vi "KG set molarity.vi"(7 "Info Cluster":T1, 8 "Fehler (Eingang, kein Fehler)":errorcluster, 9 "molarity":dbl, 10 "pump":u32, 11 "VISA-Ressourcenname":refnum<visa-resource-name>) -> (0 "Fehler (Ausgang)":errorcluster, 2 "Kommando gesendet":string, 3 "VISA-Ressourcenname (Ausgang)":refnum<visa-resource-name>)   [LabVIEW 2020, in "Linearisierung v2.lvlib" / "Gasteiler.lvlib" / "HovaCAL_Interface.lvlib" / "KGN.lvlib" / "set.lvlib"]
uses:
  set.lvlib
  Controls/Info Cluster.ctl
  KGN.lvlib
  Controls/Controls.lvlib
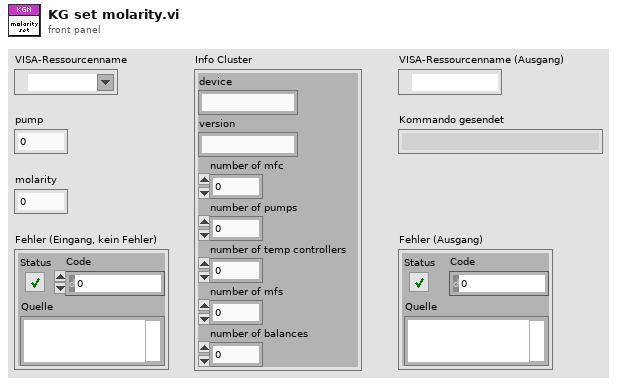
[diagram p1: front panel]
types:
  T1 = typedef "Linearisierung v2.lvlib/Gasteiler.lvlib/HovaCAL_Interface.lvlib/Controls.lvlib/Info Cluster.ctl" = cluster{"device":string, "version":string, "number of mfc":i32, "number of pumps":i32, "number of temp controllers":i32, "number of mfs":i32, "number of balances":i32}
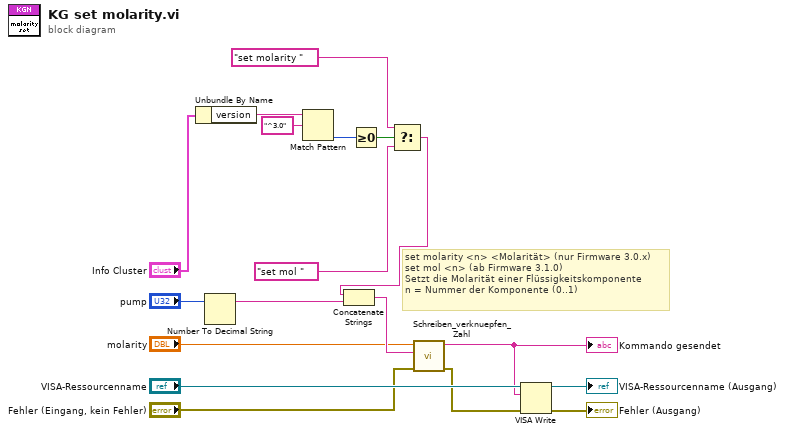
[diagram p0: block diagram]
diagram:
  # "set molarity <n> <Molarität> (nur Firmware 3.0.x)\nset mol <n> (ab Firmware 3.1.0)\nSetzt die Molarität einer Flüssigkeitskomponente\nn = Nummer der Komponente (0..1)"
  n1 = Unbundle By Name("Info Cluster") -> ("version"=w7:string)
  n2 = Number To Decimal String(number="pump") -> (decimal integer string=w14:string)  [unwired: 1 in]
  n3 = Match Pattern(string=w7, regular expression="^3.0" ("Regulärer Ausdruck")) -> (offset past match=w5:i32)  [unwired: 1 in, 3 out]
  n4 = Greater Or Equal To 0?(x=w5) -> (x >= 0?=w4:bool)
  n5 = Select(t="set molarity " ("Schreibpuffer"), s=w4, f="set mol " ("Schreibpuffer")) -> (s? t:f=w1:string)
  n6 = Concatenate Strings(w1, w14) -> (w11:string)
  n7 = call "Schreiben_verknuepfen_Zahl.vi"("error in (no error)"="Fehler (Eingang, kein Fehler)", "Order"=w11, "Zahl"="molarity") -> ("error out"=w12:errorcluster, "Verknüpfter String"=w10:string)  [unwired: 7 in]
  "Kommando gesendet" <- w10
  n8 = VISA Write(VISA resource name="VISA-Ressourcenname", write buffer=w10, error in (no error)=w12) -> (VISA resource name out=→"VISA-Ressourcenname (Ausgang)":refnum<visa-resource-name>, error out=→"Fehler (Ausgang)":errorcluster)  [unwired: 1 out]
